vi "OEE_SCREEN_1_update.vi"(8 "error_in":errorcluster) -> (0 "error_out":errorcluster, 3 "SCREEN_1":T1={"header_date"="-", "header_time"="-", "header_takt"="-", "header_shift"="-", "OP10_actual"="-", "OP10_rejects"="-", "OP10_quality_yeild"="-", "OP10_pace"="-", "OP20_actual"="-", "OP20_rejects"="-", "OP20_quality_yeild"="-", "OP20_pace"="-", "OP30_actual"="-", "OP30_rejects"="-", "OP30_quality_yeild"="-", "OP30_pace"="-", "OP40_actual"="-", "OP40_rejects"="-", "OP40_quality_yeild"="-", "OP40_pace"="-", "OP50_actual"="-", "OP50_rejects"="-", "OP50_quality_yeild"="-", "OP50_pace"="-", "OP60_actual"="-", "OP60_rejects"="-", "OP60_quality_yeild"="-", "OP60_pace"="-", "OP70_actual"="-", "OP70_rejects"="-", "OP70_quality_yeild"="-", "OP70_pace"="-", "OP80_actual"="-", "OP80_rejects"="-", "OP80_quality_yeild"="-", "OP80_pace"="-", "OP90_actual"="-", "OP90_rejects"="-", "OP90_quality_yeild"="-", "OP90_pace"="-", "OP100_actual"="-", "OP100_rejects"="-", "OP100_quality_yeild"="-", "OP100_pace"="-", "OP110_actual"="-", "OP110_rejects"="-", "OP110_quality_yeild"="-", "OP110_pace"="-", "OP120_actual"="-", "OP120_rejects"="-", "OP120_quality_yeild"="-", "OP120_pace"="-", "OP130_actual"="-", "OP130_rejects"="-", "OP130_quality_yeild"="-", "OP130_pace"="-", "OP10_header"="OP10", "OP20_header"="OP20", "OP30_header"="OP30", "OP40_header"="OP40", "OP50_header"="OP50", "OP60_header"="OP60", "OP70_header"="OP70", "OP80_header"="OP80", "OP90_header"="OP90", "OP100_header"="OP100", "OP110_header"="OP110", "OP120_header"="OP120", "OP130_header"="OP130", "additional_info"="", "bottleneck_OP"="-", "bottleneck_header"="LINE BOTTLENECK", "screen_1_header"="", "actual_header"="", "rejects_header"="", "FTTH_header"="", "pace_header"="", "actual_header"="", "rejects_header"="", "FTTH_header"="", "pace_header"=""})   [LabVIEW 2019]
uses:
  typedef/SCREEN_1.ctl
  FGV/SQL_raw_data/FGV_OEE_SQL_raw_data.ctl
panel:
  # "OP"
  # "OP"
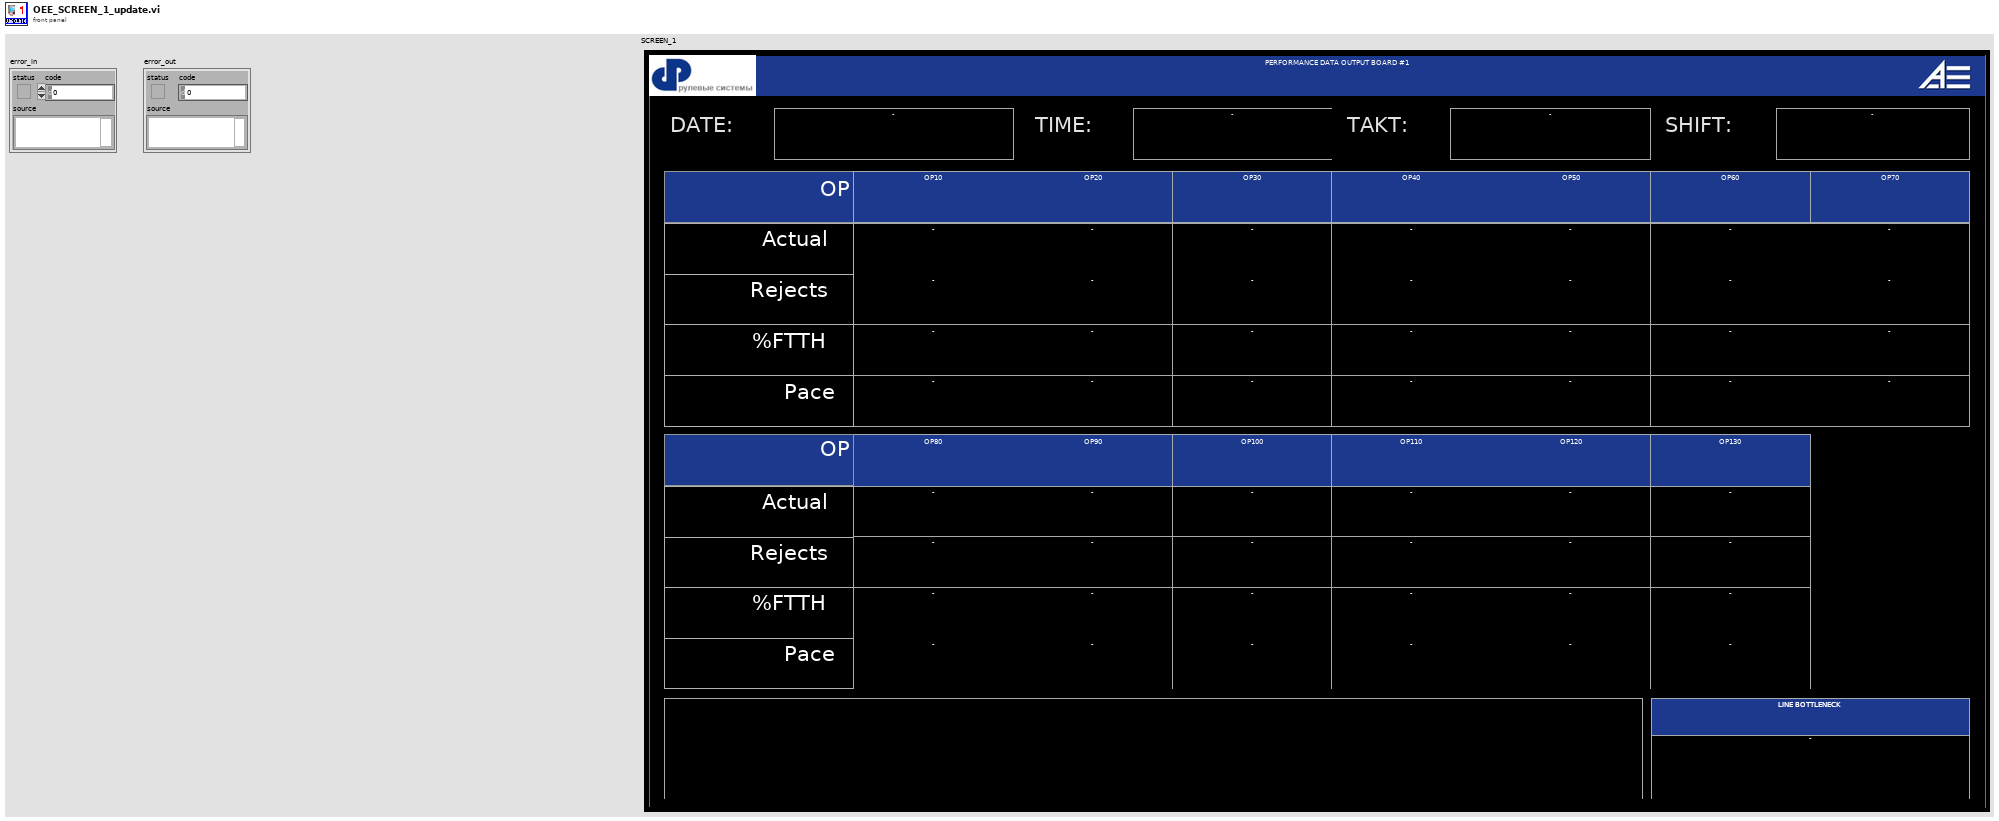
[diagram p1: front panel]
types:
  T1 = typedef "SCREEN_1.ctl" = cluster{"header_date":string, "header_time":string, "header_takt":string, "header_shift":string, "OP10_actual":string, "OP10_rejects":string, "OP10_quality_yeild":string, "OP10_pace":string, "OP20_actual":string, "OP20_rejects":string, "OP20_quality_yeild":string, "OP20_pace":string, "OP30_actual":string, "OP30_rejects":string, "OP30_quality_yeild":string, "OP30_pace":string, "OP40_actual":string, "OP40_rejects":string, "OP40_quality_yeild":string, "OP40_pace":string, "OP50_actual":string, "OP50_rejects":string, "OP50_quality_yeild":string, "OP50_pace":string, "OP60_actual":string, "OP60_rejects":string, "OP60_quality_yeild":string, "OP60_pace":string, "OP70_actual":string, "OP70_rejects":string, "OP70_quality_yeild":string, "OP70_pace":string, "OP80_actual":string, "OP80_rejects":string, "OP80_quality_yeild":string, "OP80_pace":string, "OP90_actual":string, "OP90_rejects":string, "OP90_quality_yeild":string, "OP90_pace":string, "OP100_actual":string, "OP100_rejects":string, "OP100_quality_yeild":string, "OP100_pace":string, "OP110_actual":string, "OP110_rejects":string, "OP110_quality_yeild":string, "OP110_pace":string, "OP120_actual":string, "OP120_rejects":string, "OP120_quality_yeild":string, "OP120_pace":string, "OP130_actual":string, "OP130_rejects":string, "OP130_quality_yeild":string, "OP130_pace":string, "OP10_header":string, "OP20_header":string, "OP30_header":string, "OP40_header":string, "OP50_header":string, "OP60_header":string, "OP70_header":string, "OP80_header":string, "OP90_header":string, "OP100_header":string, "OP110_header":string, "OP120_header":string, "OP130_header":string, "additional_info":string, "bottleneck_OP":string, "bottleneck_header":string, "screen_1_header":string, "actual_header":string, "rejects_header":string, "FTTH_header":string, "pace_header":string, "actual_header":string, "rejects_header":string, "FTTH_header":string, "pace_header":string}
  T2 = typedef "FGV_OEE_SQL_raw_data.ctl" = enum16{"initialize", "set_reference_name", "set_timestamp", "set_OK_NOK_count", "set_config_info", "set_pace", "set_availability", "set_hourly_ok_count", "set_targets", "get_all_info"}
  T3 = typedef "OEE_SQL_raw_data.ctl" = cluster{"reference_name":string, "data_timestamp":timestamp, "OK_NOK_count":string[][], "config_info":string[], "pace":string[][], "availability":string[], "hourly_ok_count":string[][], "shift_number":i8, "shift_start":i8, "shift_end":i8, "TAKT":u16, "FTTH_target":u16, "BOTTLENECK_station":string, "targets_hourly":u16[], "target_shift":u16}
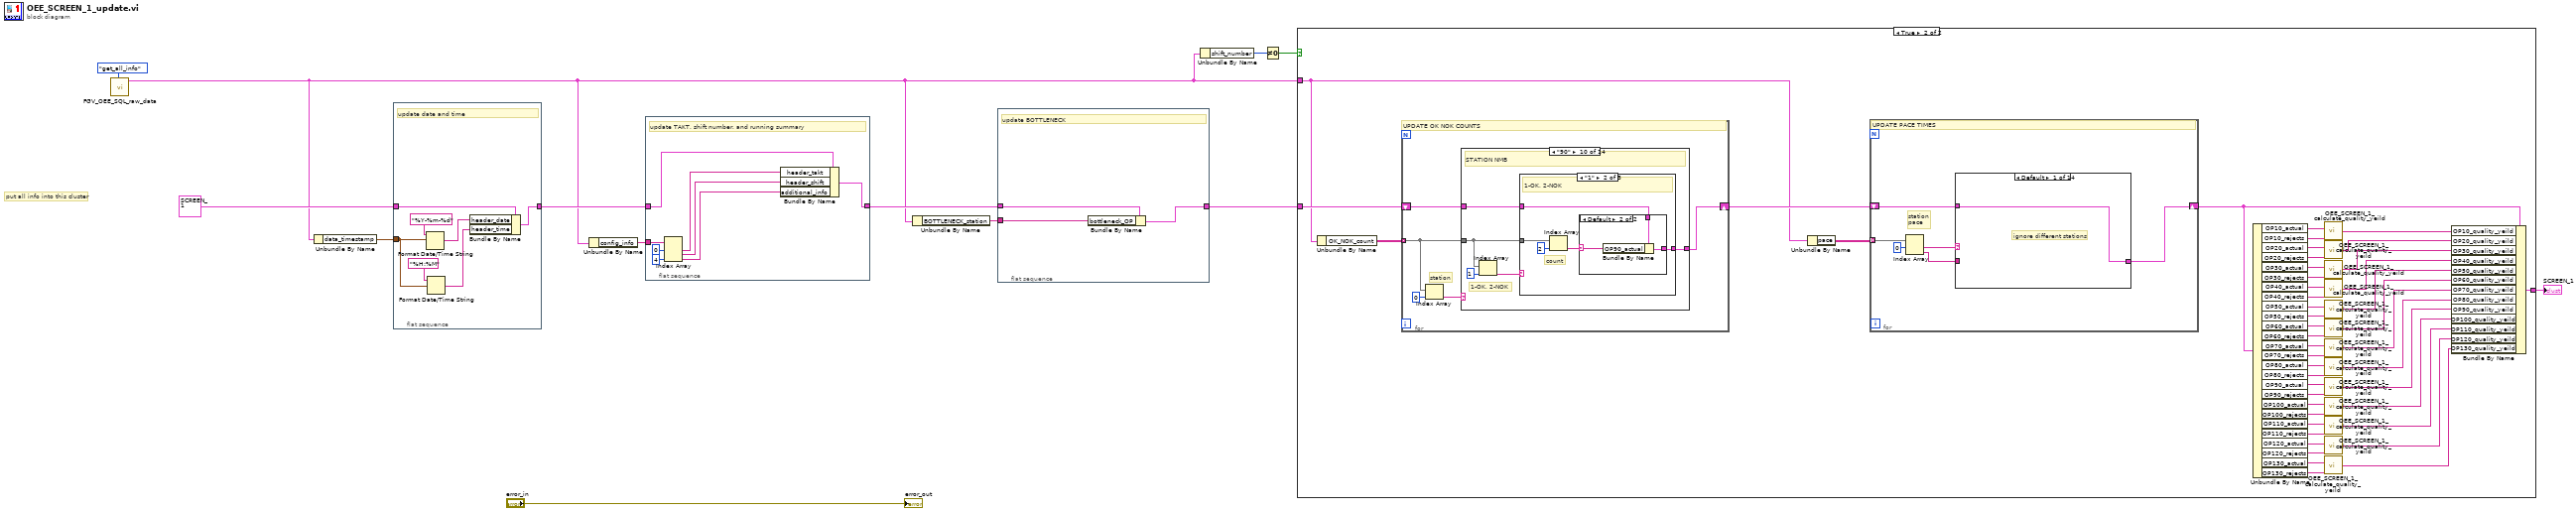
[diagram p0: block diagram]
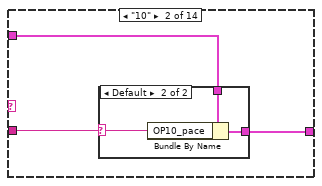
[diagram p3: hidden frame]
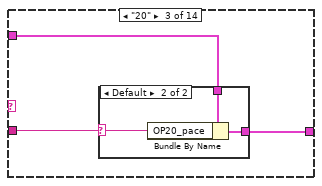
[diagram p5: hidden frame]
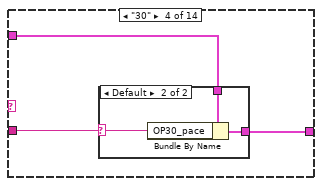
[diagram p7: hidden frame]
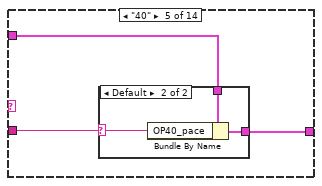
[diagram p9: hidden frame]
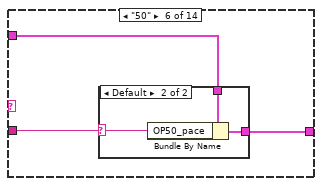
[diagram p11: hidden frame]
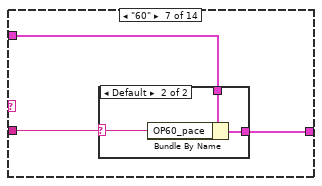
[diagram p13: hidden frame]
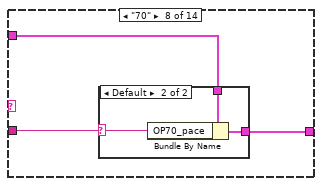
[diagram p15: hidden frame]
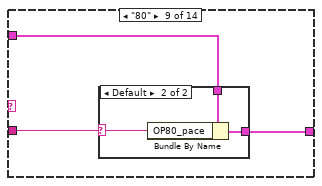
[diagram p17: hidden frame]
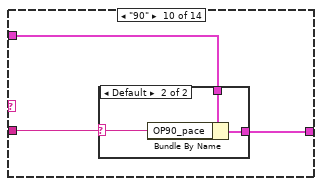
[diagram p19: hidden frame]
diagram:
  # "put all info into this cluster"
  n1 = call "FGV_OEE_SQL_raw_data.vi"("options"=FGV_OEE_SQL_raw_data."get_all_info") -> ("SQL_raw_data_out"=w3:T3)  [unwired: 9 in, 1 out]
  n2 = Unbundle By Name(w3) -> ("data_timestamp"=w8:timestamp)
  n3 = flat-sequence {
    tunnel: T1 {"header_date"="-", "header_time"="-", "header_takt"="-", "header_shift"="-", "OP10_actual"="0", "OP10_rejects"="0", "OP10_quality_yeild"="-", "OP10_pace"="-", "OP20_actual"="0", "OP20_rejects"="0", "OP20_quality_yeild"="-", "OP20_pace"="-", "OP30_actual"="0", "OP30_rejects"="0", "OP30_quality_yeild"="-", "OP30_pace"="-", "OP40_actual"="0", "OP40_rejects"="0", "OP40_quality_yeild"="-", "OP40_pace"="-", "OP50_actual"="0", "OP50_rejects"="0", "OP50_quality_yeild"="-", "OP50_pace"="-", "OP60_actual"="0", "OP60_rejects"="0", "OP60_quality_yeild"="-", "OP60_pace"="-", "OP70_actual"="0", "OP70_rejects"="0", "OP70_quality_yeild"="-", "OP70_pace"="-", "OP80_actual"="0", "OP80_rejects"="0", "OP80_quality_yeild"="-", "OP80_pace"="-", "OP90_actual"="0", "OP90_rejects"="0", "OP90_quality_yeild"="-", "OP90_pace"="-", "OP100_actual"="0", "OP100_rejects"="0", "OP100_quality_yeild"="-", "OP100_pace"="-", "OP110_actual"="0", "OP110_rejects"="0", "OP110_quality_yeild"="-", "OP110_pace"="-", "OP120_actual"="0", "OP120_rejects"="0", "OP120_quality_yeild"="-", "OP120_pace"="-", "OP130_actual"="0", "OP130_rejects"="0", "OP130_quality_yeild"="-", "OP130_pace"="-", "OP10_header"="OP10", "OP20_header"="OP20", "OP30_header"="OP30", "OP40_header"="OP40", "OP50_header"="OP50", "OP60_header"="OP60", "OP70_header"="OP70", "OP80_header"="OP80", "OP90_header"="OP90", "OP100_header"="OP100", "OP110_header"="OP110", "OP120_header"="OP120", "OP130_header"="OP130", "additional_info"="", "bottleneck_OP"="-", "bottleneck_header"="", "screen_1_header"="", "actual_header"="", "rejects_header"="", "FTTH_header"="", "pace_header"="", "actual_header"="", "rejects_header"="", "FTTH_header"="", "pace_header"=""} ("SCREEN_1") -> [w20]
    tunnel: [w19] -> w5
    tunnel: w8 -> [w15]
    frame #0 {
      # "update date and time"
      n4 = Format Date/Time String(time format string (%c)="%Y-%m-%d", seconds (now)=w15) -> (date/time string=w17:string)  [unwired: 1 in]
      n5 = Format Date/Time String(time format string (%c)="%H:%M", seconds (now)=w15) -> (date/time string=w14:string)  [unwired: 1 in]
      n6 = Bundle By Name(cluster=w20, "header_date"=w17, "header_time"=w14) -> (w19:T1)
    }
  }
  n7 = Unbundle By Name(w3) -> ("config_info"=w9:string[])
  n8 = flat-sequence {
    tunnel: w9 -> [w28]
    tunnel: w5 -> [w25]
    tunnel: [w22] -> w7
    frame #0 {
      # "update TAKT, shift number, and running summary"
      n9 = Index Array(array=w28, index #1=0 ("index"), index #3=4 ("index")) -> (element #1=w24:string, element #2=w23:string, element #3=w21:string)  [unwired: 1 in]
      n10 = Bundle By Name(cluster=w25, "header_takt"=w24, "header_shift"=w23, "additional_info"=w21) -> (w22:T1)
    }
  }
  n11 = Unbundle By Name(w3) -> ("BOTTLENECK_station"=w6:string)
  n12 = flat-sequence {
    tunnel: w7 -> [w31]
    tunnel: w6 -> [w30]
    tunnel: [w29] -> w4
    frame #0 {
      # "update BOTTLENECK"
      n13 = Bundle By Name(cluster=w31, "bottleneck_OP"=w30) -> (w29:T1)
    }
  }
  n14 = Unbundle By Name(w3) -> ("shift_number"=w1:i8)
  n15 = Not Equal To 0?(x=w1) -> (x != 0?=w2:bool)
  n16 = case shown="True" w2 {
    tunnel: [w32 w78] -> w11
    tunnel: w4 -> [w32 w35]
    tunnel: w3 -> [_ w33]
    frame False {
    }
    frame True {
      n17 = Unbundle By Name(w33) -> ("OK_NOK_count"=w77:string[][])
      n18 = for {
        tunnel: w77 -> [w180] mode=indexing
        shift-right: [w177] -> w34
        shift-left: w35 -> [w178]
        # "station"
        # "UPDATE OK NOK COUNTS"
        n19 = Index Array(array=w180, index=0) -> (element=w181:string)
        n20 = case shown="\"90\"" w181 {
          tunnel: w180 -> [_ w184 w208 w232 w256 w280 w304 w328 w352 w376 w400 w424 w448 w472]
          tunnel: w178 -> [w182 w185 w209 w233 w257 w281 w305 w329 w353 w377 w401 w425 w449 w473]
          tunnel: [w182 w183 w207 w231 w255 w279 w303 w327 w351 w375 w399 w423 w447 w471] -> w177
          frame Default {
            # "IGNORE DIFFERENT STATIONS"
          }
          frame "10" {
            # "1-OK, 2-NOK"
            # "STATION NMB"
            n21 = Index Array(array=w184, index=1) -> (element=w186:string)
            n22 = case shown="\"1\"" w186 {
              tunnel: w185 -> [w188 w193 w202]
              tunnel: w184 -> [_ w192 w201]
              tunnel: [w188 w189 w198] -> w183
              frame Default {
                # "IGNORE DIFFERENT VALUES"
              }
              frame "1" {
                # "count"
                # "1-OK, 2-NOK"
                n23 = Index Array(array=w192, index=2) -> (element=w190:string)
                n24 = case shown="Default" w190 {
                  selector: w190 -> [_ w196]
                  tunnel: w193 -> [w194 w197]
                  tunnel: [w194 w195] -> w189
                  frame "" {
                    # "ignore NULLs"
                  }
                  frame Default {
                    n25 = Bundle By Name(cluster=w197, "OP10_actual"=w196) -> (w195:T1)
                  }
                }
              }
              frame "2" {
                # "count"
                # "1-OK, 2-NOK"
                n26 = Index Array(array=w201, index=2) -> (element=w199:string)
                n27 = case shown="Default" w199 {
                  selector: w199 -> [_ w205]
                  tunnel: w202 -> [w203 w206]
                  tunnel: [w203 w204] -> w198
                  frame "" {
                    # "ignore NULLs"
                  }
                  frame Default {
                    n28 = Bundle By Name(cluster=w206, "OP10_rejects"=w205) -> (w204:T1)
                  }
                }
              }
            }
          }
          frame "20" {
            # "1-OK, 2-NOK"
            # "STATION NMB"
            n29 = Index Array(array=w208, index=1) -> (element=w210:string)
            n30 = case shown="\"1\"" w210 {
              tunnel: w209 -> [w212 w217 w226]
              tunnel: w208 -> [_ w216 w225]
              tunnel: [w212 w213 w222] -> w207
              frame Default {
                # "IGNORE DIFFERENT VALUES"
              }
              frame "1" {
                # "count"
                # "1-OK, 2-NOK"
                n31 = Index Array(array=w216, index=2) -> (element=w214:string)
                n32 = case shown="Default" w214 {
                  selector: w214 -> [_ w220]
                  tunnel: w217 -> [w218 w221]
                  tunnel: [w218 w219] -> w213
                  frame "" {
                    # "ignore NULLs"
                  }
                  frame Default {
                    n33 = Bundle By Name(cluster=w221, "OP20_actual"=w220) -> (w219:T1)
                  }
                }
              }
              frame "2" {
                # "count"
                # "1-OK, 2-NOK"
                n34 = Index Array(array=w225, index=2) -> (element=w223:string)
                n35 = case shown="Default" w223 {
                  selector: w223 -> [_ w229]
                  tunnel: w226 -> [w227 w230]
                  tunnel: [w227 w228] -> w222
                  frame "" {
                    # "ignore NULLs"
                  }
                  frame Default {
                    n36 = Bundle By Name(cluster=w230, "OP20_rejects"=w229) -> (w228:T1)
                  }
                }
              }
            }
          }
          frame "30" {
            # "1-OK, 2-NOK"
            # "STATION NMB"
            n37 = Index Array(array=w232, index=1) -> (element=w234:string)
            n38 = case shown="\"1\"" w234 {
              tunnel: w233 -> [w236 w241 w250]
              tunnel: w232 -> [_ w240 w249]
              tunnel: [w236 w237 w246] -> w231
              frame Default {
                # "IGNORE DIFFERENT VALUES"
              }
              frame "1" {
                # "count"
                # "1-OK, 2-NOK"
                n39 = Index Array(array=w240, index=2) -> (element=w238:string)
                n40 = case shown="Default" w238 {
                  selector: w238 -> [_ w244]
                  tunnel: w241 -> [w242 w245]
                  tunnel: [w242 w243] -> w237
                  frame "" {
                    # "ignore NULLs"
                  }
                  frame Default {
                    n41 = Bundle By Name(cluster=w245, "OP30_actual"=w244) -> (w243:T1)
                  }
                }
              }
              frame "2" {
                # "count"
                # "1-OK, 2-NOK"
                n42 = Index Array(array=w249, index=2) -> (element=w247:string)
                n43 = case shown="Default" w247 {
                  selector: w247 -> [_ w253]
                  tunnel: w250 -> [w251 w254]
                  tunnel: [w251 w252] -> w246
                  frame "" {
                    # "ignore NULLs"
                  }
                  frame Default {
                    n44 = Bundle By Name(cluster=w254, "OP30_rejects"=w253) -> (w252:T1)
                  }
                }
              }
            }
          }
          frame "40" {
            # "1-OK, 2-NOK"
            # "STATION NMB"
            n45 = Index Array(array=w256, index=1) -> (element=w258:string)
            n46 = case shown="\"1\"" w258 {
              tunnel: w257 -> [w260 w265 w274]
              tunnel: w256 -> [_ w264 w273]
              tunnel: [w260 w261 w270] -> w255
              frame Default {
                # "IGNORE DIFFERENT VALUES"
              }
              frame "1" {
                # "count"
                # "1-OK, 2-NOK"
                n47 = Index Array(array=w264, index=2) -> (element=w262:string)
                n48 = case shown="Default" w262 {
                  selector: w262 -> [_ w268]
                  tunnel: w265 -> [w266 w269]
                  tunnel: [w266 w267] -> w261
                  frame "" {
                    # "ignore NULLs"
                  }
                  frame Default {
                    n49 = Bundle By Name(cluster=w269, "OP40_actual"=w268) -> (w267:T1)
                  }
                }
              }
              frame "2" {
                # "count"
                # "1-OK, 2-NOK"
                n50 = Index Array(array=w273, index=2) -> (element=w271:string)
                n51 = case shown="Default" w271 {
                  selector: w271 -> [_ w277]
                  tunnel: w274 -> [w275 w278]
                  tunnel: [w275 w276] -> w270
                  frame "" {
                    # "ignore NULLs"
                  }
                  frame Default {
                    n52 = Bundle By Name(cluster=w278, "OP40_rejects"=w277) -> (w276:T1)
                  }
                }
              }
            }
          }
          frame "50" {
            # "1-OK, 2-NOK"
            # "STATION NMB"
            n53 = Index Array(array=w280, index=1) -> (element=w282:string)
            n54 = case shown="\"1\"" w282 {
              tunnel: w281 -> [w284 w289 w298]
              tunnel: w280 -> [_ w288 w297]
              tunnel: [w284 w285 w294] -> w279
              frame Default {
                # "IGNORE DIFFERENT VALUES"
              }
              frame "1" {
                # "count"
                # "1-OK, 2-NOK"
                n55 = Index Array(array=w288, index=2) -> (element=w286:string)
                n56 = case shown="Default" w286 {
                  selector: w286 -> [_ w292]
                  tunnel: w289 -> [w290 w293]
                  tunnel: [w290 w291] -> w285
                  frame "" {
                    # "ignore NULLs"
                  }
                  frame Default {
                    n57 = Bundle By Name(cluster=w293, "OP50_actual"=w292) -> (w291:T1)
                  }
                }
              }
              frame "2" {
                # "count"
                # "1-OK, 2-NOK"
                n58 = Index Array(array=w297, index=2) -> (element=w295:string)
                n59 = case shown="Default" w295 {
                  selector: w295 -> [_ w301]
                  tunnel: w298 -> [w299 w302]
                  tunnel: [w299 w300] -> w294
                  frame "" {
                    # "ignore NULLs"
                  }
                  frame Default {
                    n60 = Bundle By Name(cluster=w302, "OP50_rejects"=w301) -> (w300:T1)
                  }
                }
              }
            }
          }
          frame "60" {
            # "1-OK, 2-NOK"
            # "STATION NMB"
            n61 = Index Array(array=w304, index=1) -> (element=w306:string)
            n62 = case shown="\"1\"" w306 {
              tunnel: w305 -> [w308 w313 w322]
              tunnel: w304 -> [_ w312 w321]
              tunnel: [w308 w309 w318] -> w303
              frame Default {
                # "IGNORE DIFFERENT VALUES"
              }
              frame "1" {
                # "count"
                # "1-OK, 2-NOK"
                n63 = Index Array(array=w312, index=2) -> (element=w310:string)
                n64 = case shown="Default" w310 {
                  selector: w310 -> [_ w316]
                  tunnel: w313 -> [w314 w317]
                  tunnel: [w314 w315] -> w309
                  frame "" {
                    # "ignore NULLs"
                  }
                  frame Default {
                    n65 = Bundle By Name(cluster=w317, "OP60_actual"=w316) -> (w315:T1)
                  }
                }
              }
              frame "2" {
                # "count"
                # "1-OK, 2-NOK"
                n66 = Index Array(array=w321, index=2) -> (element=w319:string)
                n67 = case shown="Default" w319 {
                  selector: w319 -> [_ w325]
                  tunnel: w322 -> [w323 w326]
                  tunnel: [w323 w324] -> w318
                  frame "" {
                    # "ignore NULLs"
                  }
                  frame Default {
                    n68 = Bundle By Name(cluster=w326, "OP60_rejects"=w325) -> (w324:T1)
                  }
                }
              }
            }
          }
          frame "70" {
            # "1-OK, 2-NOK"
            # "STATION NMB"
            n69 = Index Array(array=w328, index=1) -> (element=w330:string)
            n70 = case shown="\"1\"" w330 {
              tunnel: w329 -> [w332 w337 w346]
              tunnel: w328 -> [_ w336 w345]
              tunnel: [w332 w333 w342] -> w327
              frame Default {
                # "IGNORE DIFFERENT VALUES"
              }
              frame "1" {
                # "count"
                # "1-OK, 2-NOK"
                n71 = Index Array(array=w336, index=2) -> (element=w334:string)
                n72 = case shown="Default" w334 {
                  selector: w334 -> [_ w340]
                  tunnel: w337 -> [w338 w341]
                  tunnel: [w338 w339] -> w333
                  frame "" {
                    # "ignore NULLs"
                  }
                  frame Default {
                    n73 = Bundle By Name(cluster=w341, "OP70_actual"=w340) -> (w339:T1)
                  }
                }
              }
              frame "2" {
                # "count"
                # "1-OK, 2-NOK"
                n74 = Index Array(array=w345, index=2) -> (element=w343:string)
                n75 = case shown="Default" w343 {
                  selector: w343 -> [_ w349]
                  tunnel: w346 -> [w347 w350]
                  tunnel: [w347 w348] -> w342
                  frame "" {
                    # "ignore NULLs"
                  }
                  frame Default {
                    n76 = Bundle By Name(cluster=w350, "OP70_rejects"=w349) -> (w348:T1)
                  }
                }
              }
            }
          }
          frame "80" {
            # "1-OK, 2-NOK"
            # "STATION NMB"
            n77 = Index Array(array=w352, index=1) -> (element=w354:string)
            n78 = case shown="\"1\"" w354 {
              tunnel: w353 -> [w356 w361 w370]
              tunnel: w352 -> [_ w360 w369]
              tunnel: [w356 w357 w366] -> w351
              frame Default {
                # "IGNORE DIFFERENT VALUES"
              }
              frame "1" {
                # "count"
                # "1-OK, 2-NOK"
                n79 = Index Array(array=w360, index=2) -> (element=w358:string)
                n80 = case shown="Default" w358 {
                  selector: w358 -> [_ w364]
                  tunnel: w361 -> [w362 w365]
                  tunnel: [w362 w363] -> w357
                  frame "" {
                    # "ignore NULLs"
                  }
                  frame Default {
                    n81 = Bundle By Name(cluster=w365, "OP80_actual"=w364) -> (w363:T1)
                  }
                }
              }
              frame "2" {
                # "count"
                # "1-OK, 2-NOK"
                n82 = Index Array(array=w369, index=2) -> (element=w367:string)
                n83 = case shown="Default" w367 {
                  selector: w367 -> [_ w373]
                  tunnel: w370 -> [w371 w374]
                  tunnel: [w371 w372] -> w366
                  frame "" {
                    # "ignore NULLs"
                  }
                  frame Default {
                    n84 = Bundle By Name(cluster=w374, "OP80_rejects"=w373) -> (w372:T1)
                  }
                }
              }
            }
          }
          frame "90" {
            # "1-OK, 2-NOK"
            # "STATION NMB"
            n85 = Index Array(array=w376, index=1) -> (element=w378:string)
            n86 = case shown="\"1\"" w378 {
              tunnel: w377 -> [w380 w385 w394]
              tunnel: w376 -> [_ w384 w393]
              tunnel: [w380 w381 w390] -> w375
              frame Default {
                # "IGNORE DIFFERENT VALUES"
              }
              frame "1" {
                # "count"
                # "1-OK, 2-NOK"
                n87 = Index Array(array=w384, index=2) -> (element=w382:string)
                n88 = case shown="Default" w382 {
                  selector: w382 -> [_ w388]
                  tunnel: w385 -> [w386 w389]
                  tunnel: [w386 w387] -> w381
                  frame "" {
                    # "ignore NULLs"
                  }
                  frame Default {
                    n89 = Bundle By Name(cluster=w389, "OP90_actual"=w388) -> (w387:T1)
                  }
                }
              }
              frame "2" {
                # "count"
                # "1-OK, 2-NOK"
                n90 = Index Array(array=w393, index=2) -> (element=w391:string)
                n91 = case shown="Default" w391 {
                  selector: w391 -> [_ w397]
                  tunnel: w394 -> [w395 w398]
                  tunnel: [w395 w396] -> w390
                  frame "" {
                    # "ignore NULLs"
                  }
                  frame Default {
                    n92 = Bundle By Name(cluster=w398, "OP90_rejects"=w397) -> (w396:T1)
                  }
                }
              }
            }
          }
          frame "100" {
            # "1-OK, 2-NOK"
            # "STATION NMB"
            n93 = Index Array(array=w400, index=1) -> (element=w402:string)
            n94 = case shown="\"1\"" w402 {
              tunnel: w401 -> [w404 w409 w418]
              tunnel: w400 -> [_ w408 w417]
              tunnel: [w404 w405 w414] -> w399
              frame Default {
                # "IGNORE DIFFERENT VALUES"
              }
              frame "1" {
                # "count"
                # "1-OK, 2-NOK"
                n95 = Index Array(array=w408, index=2) -> (element=w406:string)
                n96 = case shown="Default" w406 {
                  selector: w406 -> [_ w412]
                  tunnel: w409 -> [w410 w413]
                  tunnel: [w410 w411] -> w405
                  frame "" {
                    # "ignore NULLs"
                  }
                  frame Default {
                    n97 = Bundle By Name(cluster=w413, "OP100_actual"=w412) -> (w411:T1)
                  }
                }
              }
              frame "2" {
                # "count"
                # "1-OK, 2-NOK"
                n98 = Index Array(array=w417, index=2) -> (element=w415:string)
                n99 = case shown="Default" w415 {
                  selector: w415 -> [_ w421]
                  tunnel: w418 -> [w419 w422]
                  tunnel: [w419 w420] -> w414
                  frame "" {
                    # "ignore NULLs"
                  }
                  frame Default {
                    n100 = Bundle By Name(cluster=w422, "OP100_rejects"=w421) -> (w420:T1)
                  }
                }
              }
            }
          }
          frame "110" {
            # "1-OK, 2-NOK"
            # "STATION NMB"
            n101 = Index Array(array=w424, index=1) -> (element=w426:string)
            n102 = case shown="\"1\"" w426 {
              tunnel: w425 -> [w428 w433 w442]
              tunnel: w424 -> [_ w432 w441]
              tunnel: [w428 w429 w438] -> w423
              frame Default {
                # "IGNORE DIFFERENT VALUES"
              }
              frame "1" {
                # "count"
                # "1-OK, 2-NOK"
                n103 = Index Array(array=w432, index=2) -> (element=w430:string)
                n104 = case shown="Default" w430 {
                  selector: w430 -> [_ w436]
                  tunnel: w433 -> [w434 w437]
                  tunnel: [w434 w435] -> w429
                  frame "" {
                    # "ignore NULLs"
                  }
                  frame Default {
                    n105 = Bundle By Name(cluster=w437, "OP110_actual"=w436) -> (w435:T1)
                  }
                }
              }
              frame "2" {
                # "count"
                # "1-OK, 2-NOK"
                n106 = Index Array(array=w441, index=2) -> (element=w439:string)
                n107 = case shown="Default" w439 {
                  selector: w439 -> [_ w445]
                  tunnel: w442 -> [w443 w446]
                  tunnel: [w443 w444] -> w438
                  frame "" {
                    # "ignore NULLs"
                  }
                  frame Default {
                    n108 = Bundle By Name(cluster=w446, "OP110_rejects"=w445) -> (w444:T1)
                  }
                }
              }
            }
          }
          frame "120" {
            # "1-OK, 2-NOK"
            # "STATION NMB"
            n109 = Index Array(array=w448, index=1) -> (element=w450:string)
            n110 = case shown="\"1\"" w450 {
              tunnel: w449 -> [w452 w457 w466]
              tunnel: w448 -> [_ w456 w465]
              tunnel: [w452 w453 w462] -> w447
              frame Default {
                # "IGNORE DIFFERENT VALUES"
              }
              frame "1" {
                # "count"
                # "1-OK, 2-NOK"
                n111 = Index Array(array=w456, index=2) -> (element=w454:string)
                n112 = case shown="Default" w454 {
                  selector: w454 -> [_ w460]
                  tunnel: w457 -> [w458 w461]
                  tunnel: [w458 w459] -> w453
                  frame "" {
                    # "ignore NULLs"
                  }
                  frame Default {
                    n113 = Bundle By Name(cluster=w461, "OP120_actual"=w460) -> (w459:T1)
                  }
                }
              }
              frame "2" {
                # "count"
                # "1-OK, 2-NOK"
                n114 = Index Array(array=w465, index=2) -> (element=w463:string)
                n115 = case shown="Default" w463 {
                  selector: w463 -> [_ w469]
                  tunnel: w466 -> [w467 w470]
                  tunnel: [w467 w468] -> w462
                  frame "" {
                    # "ignore NULLs"
                  }
                  frame Default {
                    n116 = Bundle By Name(cluster=w470, "OP120_rejects"=w469) -> (w468:T1)
                  }
                }
              }
            }
          }
          frame "130" {
            # "1-OK, 2-NOK"
            # "STATION NMB"
            n117 = Index Array(array=w472, index=1) -> (element=w474:string)
            n118 = case shown="\"1\"" w474 {
              tunnel: w473 -> [w476 w481 w490]
              tunnel: w472 -> [_ w480 w489]
              tunnel: [w476 w477 w486] -> w471
              frame Default {
                # "IGNORE DIFFERENT VALUES"
              }
              frame "1" {
                # "count"
                # "1-OK, 2-NOK"
                n119 = Index Array(array=w480, index=2) -> (element=w478:string)
                n120 = case shown="Default" w478 {
                  selector: w478 -> [_ w484]
                  tunnel: w481 -> [w482 w485]
                  tunnel: [w482 w483] -> w477
                  frame "" {
                    # "ignore NULLs"
                  }
                  frame Default {
                    n121 = Bundle By Name(cluster=w485, "OP130_actual"=w484) -> (w483:T1)
                  }
                }
              }
              frame "2" {
                # "count"
                # "1-OK, 2-NOK"
                n122 = Index Array(array=w489, index=2) -> (element=w487:string)
                n123 = case shown="Default" w487 {
                  selector: w487 -> [_ w493]
                  tunnel: w490 -> [w491 w494]
                  tunnel: [w491 w492] -> w486
                  frame "" {
                    # "ignore NULLs"
                  }
                  frame Default {
                    n124 = Bundle By Name(cluster=w494, "OP130_rejects"=w493) -> (w492:T1)
                  }
                }
              }
            }
          }
        }
      }
      n125 = Unbundle By Name(w33) -> ("pace"=w37:string[][])
      n126 = for {
        tunnel: w37 -> [w84] mode=indexing
        shift-right: [w82] -> w36
        shift-left: w34 -> [w81]
        # "station\npace"
        # "UPDATE PACE TIMES"
        n127 = Index Array(array=w84, index #1=0 ("index")) -> (element #1=w79:string, element #2=w80:string)  [unwired: 1 in]
        n128 = case shown="Default" w79 {
          tunnel: [w85 w88 w95 w102 w109 w116 w123 w130 w137 w144 w151 w158 w165 w172] -> w82
          tunnel: w81 -> [w85 w87 w94 w101 w108 w115 w122 w129 w136 w143 w150 w157 w164 w171]
          tunnel: w80 -> [_ w86 w93 w100 w107 w114 w121 w128 w135 w142 w149 w156 w163 w170]
          frame Default {
            # "ignore different stations"
          }
          frame "10" {
            n129 = case shown="Default" w86 {
              selector: w86 -> [_ w91]
              tunnel: w87 -> [w89 w92]
              tunnel: [w89 w90] -> w88
              frame "" {
                # "ignore NULLs"
              }
              frame Default {
                n130 = Bundle By Name(cluster=w92, "OP10_pace"=w91) -> (w90:T1)
              }
            }
          }
          frame "20" {
            n131 = case shown="Default" w93 {
              selector: w93 -> [_ w98]
              tunnel: w94 -> [w96 w99]
              tunnel: [w96 w97] -> w95
              frame "" {
                # "ignore NULLs"
              }
              frame Default {
                n132 = Bundle By Name(cluster=w99, "OP20_pace"=w98) -> (w97:T1)
              }
            }
          }
          frame "30" {
            n133 = case shown="Default" w100 {
              selector: w100 -> [_ w105]
              tunnel: w101 -> [w103 w106]
              tunnel: [w103 w104] -> w102
              frame "" {
                # "ignore NULLs"
              }
              frame Default {
                n134 = Bundle By Name(cluster=w106, "OP30_pace"=w105) -> (w104:T1)
              }
            }
          }
          frame "40" {
            n135 = case shown="Default" w107 {
              selector: w107 -> [_ w112]
              tunnel: w108 -> [w110 w113]
              tunnel: [w110 w111] -> w109
              frame "" {
                # "ignore NULLs"
              }
              frame Default {
                n136 = Bundle By Name(cluster=w113, "OP40_pace"=w112) -> (w111:T1)
              }
            }
          }
          frame "50" {
            n137 = case shown="Default" w114 {
              selector: w114 -> [_ w119]
              tunnel: w115 -> [w117 w120]
              tunnel: [w117 w118] -> w116
              frame "" {
                # "ignore NULLs"
              }
              frame Default {
                n138 = Bundle By Name(cluster=w120, "OP50_pace"=w119) -> (w118:T1)
              }
            }
          }
          frame "60" {
            n139 = case shown="Default" w121 {
              selector: w121 -> [_ w126]
              tunnel: w122 -> [w124 w127]
              tunnel: [w124 w125] -> w123
              frame "" {
                # "ignore NULLs"
              }
              frame Default {
                n140 = Bundle By Name(cluster=w127, "OP60_pace"=w126) -> (w125:T1)
              }
            }
          }
          frame "70" {
            n141 = case shown="Default" w128 {
              selector: w128 -> [_ w133]
              tunnel: w129 -> [w131 w134]
              tunnel: [w131 w132] -> w130
              frame "" {
                # "ignore NULLs"
              }
              frame Default {
                n142 = Bundle By Name(cluster=w134, "OP70_pace"=w133) -> (w132:T1)
              }
            }
          }
          frame "80" {
            n143 = case shown="Default" w135 {
              selector: w135 -> [_ w140]
              tunnel: w136 -> [w138 w141]
              tunnel: [w138 w139] -> w137
              frame "" {
                # "ignore NULLs"
              }
              frame Default {
                n144 = Bundle By Name(cluster=w141, "OP80_pace"=w140) -> (w139:T1)
              }
            }
          }
          frame "90" {
            n145 = case shown="Default" w142 {
              selector: w142 -> [_ w147]
              tunnel: w143 -> [w145 w148]
              tunnel: [w145 w146] -> w144
              frame "" {
                # "ignore NULLs"
              }
              frame Default {
                n146 = Bundle By Name(cluster=w148, "OP90_pace"=w147) -> (w146:T1)
              }
            }
          }
          frame "100" {
            n147 = case shown="Default" w149 {
              selector: w149 -> [_ w154]
              tunnel: w150 -> [w152 w155]
              tunnel: [w152 w153] -> w151
              frame "" {
                # "ignore NULLs"
              }
              frame Default {
                n148 = Bundle By Name(cluster=w155, "OP100_pace"=w154) -> (w153:T1)
              }
            }
          }
          frame "110" {
            n149 = case shown="Default" w156 {
              selector: w156 -> [_ w161]
              tunnel: w157 -> [w159 w162]
              tunnel: [w159 w160] -> w158
              frame "" {
                # "ignore NULLs"
              }
              frame Default {
                n150 = Bundle By Name(cluster=w162, "OP110_pace"=w161) -> (w160:T1)
              }
            }
          }
          frame "120" {
            n151 = case shown="Default" w163 {
              selector: w163 -> [_ w168]
              tunnel: w164 -> [w166 w169]
              tunnel: [w166 w167] -> w165
              frame "" {
                # "ignore NULLs"
              }
              frame Default {
                n152 = Bundle By Name(cluster=w169, "OP120_pace"=w168) -> (w167:T1)
              }
            }
          }
          frame "130" {
            n153 = case shown="Default" w170 {
              selector: w170 -> [_ w175]
              tunnel: w171 -> [w173 w176]
              tunnel: [w173 w174] -> w172
              frame "" {
                # "ignore NULLs"
              }
              frame Default {
                n154 = Bundle By Name(cluster=w176, "OP130_pace"=w175) -> (w174:T1)
              }
            }
          }
        }
      }
      n155 = Unbundle By Name(w36) -> ("OP10_actual"=w76:string, "OP10_rejects"=w75:string, "OP20_actual"=w73:string, "OP20_rejects"=w72:string, "OP30_actual"=w71:string, "OP30_rejects"=w70:string, "OP40_actual"=w69:string, "OP40_rejects"=w68:string, "OP50_actual"=w67:string, "OP50_rejects"=w66:string, "OP60_actual"=w65:string, "OP60_rejects"=w64:string, "OP70_actual"=w63:string, "OP70_rejects"=w62:string, "OP80_actual"=w61:string, "OP80_rejects"=w60:string, "OP90_actual"=w59:string, "OP90_rejects"=w58:string, "OP100_actual"=w57:string, "OP100_rejects"=w56:string, "OP110_actual"=w55:string, "OP110_rejects"=w54:string, "OP120_actual"=w53:string, "OP120_rejects"=w52:string, "OP130_actual"=w51:string, "OP130_rejects"=w50:string)
      n156 = call "OEE_SCREEN_1_calculate_quality_yeild.vi"("rejects"=w75, "actual"=w76) -> ("quality_yeild"=w74:string)  [unwired: 2 in]
      n157 = call "OEE_SCREEN_1_calculate_quality_yeild.vi"("rejects"=w72, "actual"=w73) -> ("quality_yeild"=w49:string)  [unwired: 2 in]
      n158 = call "OEE_SCREEN_1_calculate_quality_yeild.vi"("rejects"=w70, "actual"=w71) -> ("quality_yeild"=w48:string)  [unwired: 2 in]
      n159 = call "OEE_SCREEN_1_calculate_quality_yeild.vi"("rejects"=w68, "actual"=w69) -> ("quality_yeild"=w47:string)  [unwired: 2 in]
      n160 = call "OEE_SCREEN_1_calculate_quality_yeild.vi"("rejects"=w66, "actual"=w67) -> ("quality_yeild"=w46:string)  [unwired: 2 in]
      n161 = call "OEE_SCREEN_1_calculate_quality_yeild.vi"("rejects"=w64, "actual"=w65) -> ("quality_yeild"=w45:string)  [unwired: 2 in]
      n162 = call "OEE_SCREEN_1_calculate_quality_yeild.vi"("rejects"=w62, "actual"=w63) -> ("quality_yeild"=w44:string)  [unwired: 2 in]
      n163 = call "OEE_SCREEN_1_calculate_quality_yeild.vi"("rejects"=w60, "actual"=w61) -> ("quality_yeild"=w43:string)  [unwired: 2 in]
      n164 = call "OEE_SCREEN_1_calculate_quality_yeild.vi"("rejects"=w58, "actual"=w59) -> ("quality_yeild"=w42:string)  [unwired: 2 in]
      n165 = call "OEE_SCREEN_1_calculate_quality_yeild.vi"("rejects"=w56, "actual"=w57) -> ("quality_yeild"=w41:string)  [unwired: 2 in]
      n166 = call "OEE_SCREEN_1_calculate_quality_yeild.vi"("rejects"=w54, "actual"=w55) -> ("quality_yeild"=w40:string)  [unwired: 2 in]
      n167 = call "OEE_SCREEN_1_calculate_quality_yeild.vi"("rejects"=w52, "actual"=w53) -> ("quality_yeild"=w39:string)  [unwired: 2 in]
      n168 = call "OEE_SCREEN_1_calculate_quality_yeild.vi"("rejects"=w50, "actual"=w51) -> ("quality_yeild"=w38:string)  [unwired: 2 in]
      n169 = Bundle By Name(cluster=w36, "OP10_quality_yeild"=w74, "OP20_quality_yeild"=w49, "OP30_quality_yeild"=w48, "OP40_quality_yeild"=w47, "OP50_quality_yeild"=w46, "OP60_quality_yeild"=w45, "OP70_quality_yeild"=w44, "OP80_quality_yeild"=w43, "OP90_quality_yeild"=w42, "OP100_quality_yeild"=w41, "OP110_quality_yeild"=w40, "OP120_quality_yeild"=w39, "OP130_quality_yeild"=w38) -> (w78:T1)
    }
  }
  "SCREEN_1" <- w11
  "error_out" <- "error_in"
